vi "EdgeTrigger.vi"(0 "Input Signal":bool) -> (1 "Rising Edge Trigger":bool, 2 "All Edge Trigger":bool, 3 "Falling Edge Trigger":bool)   [LabVIEW 2018]
doc: "This VI detects rising and falling edges of boolean inputs and also outputs whenever any edge is detected."
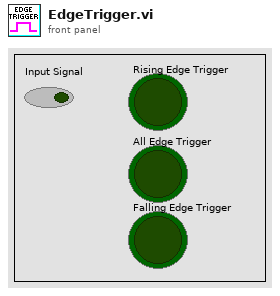
[diagram p1: front panel]
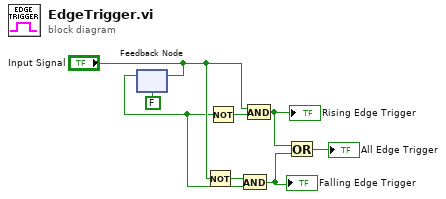
[diagram p0: block diagram]
diagram:
  n1 = feedback #1(FALSE ("Button")) -> (w4:bool)
  n2 = feedback-in #1("Input Signal") -> ()
  n3 = Not(x="Input Signal") -> (.not. x?=w5:bool)
  n4 = Not(x=w4) -> (.not. x?=w8:bool)
  n5 = And(x=w5, y=w4) -> (x .and. y?=w2:bool)
  "Falling Edge Trigger" <- w2
  n6 = And(x="Input Signal", y=w8) -> (x .and. y?=w3:bool)
  "Rising Edge Trigger" <- w3
  n7 = Or(x=w3, y=w2) -> (x .or. y?=→"All Edge Trigger":bool)
